vi "IMAQDevice.get_VideoModesAndAttributes.vi"(0 "i ref in":refnum<vi>, 5 "error in (no error)":errorcluster) -> (14 "i ref out":refnum<vi>, 16 "Video Modes":T3(array[cluster]), 17 "Attribute Information":T2(array[cluster]), 18 "Attribute Names":string[](array[string]), 19 "error out":errorcluster)   [LabVIEW 2014, in "IMAQDevice.lvlib"]
doc: "This VI reads back information from the camera.\n\nLicense Agreement for this software:\n\nCopyright (C)\nGesellschaft für Schwerionenforschung, GSI\nPlanckstr. 1\n64291 Darmstadt\nGermany\n\nContact: D.Beck@gsi.de \n\nThis program is free software; you can redistribute it and/or modify it under the terms of the \nGNU General Public License as published by the Free Software Foundation; either version 2 of \nthe license, or (at your option) any later version.\n\nThis program is distributed in the hope that it will be useful, but WITHOUT ANY WARRANTY; \nwithout even the implied warranty of MERCHANTABILITY or FITNESS FOR A PARTICULAR PURPOSE. See the GNU General License for more details (http://www.gnu.org).\n\nGesellschaft für Schwerionenforschung, GSI\nPlanckstr. 1, 64291 Darmstadt, Germany\nFor all questions and ideas contact: M.Richter@gsi.de, H.Brand@gsi.de or D.Beck@gsi.de.\nLast update: 16-JUN-2004"
uses:
  IMAQDevice.lvlib
  CSlibraries-extern/HGF/HGF_LVC/HGF_IMAQ/HGF_IMAQDevice/HGF_IMAQDevice.lvclass
  <vilib>/vision/driver/IMAQdx.llb/IMAQdx Attribute Type.ctl
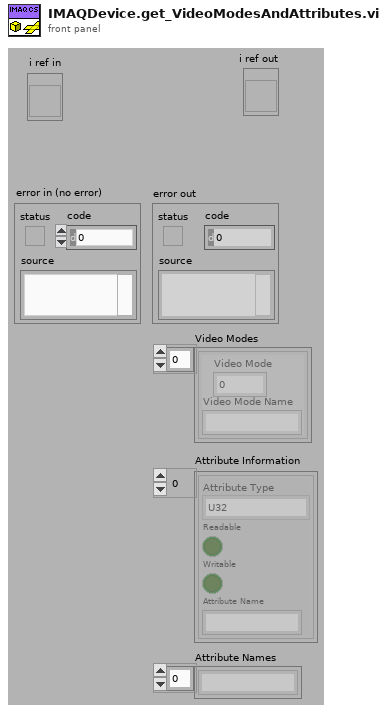
[diagram p1: front panel]
types:
  T1 = typedef "NI_Vision_Acquisition_Software.lvlib/IMAQdx Attribute Type.ctl" = enum32{"U32", "I64", "DBL", "String", "Enum", "Bool", "Command"}
  T2 = cluster{"Attribute Type":T1, "Readable":bool, "Writable":bool, "Attribute Name":string}[]
  T3 = cluster{"Video Mode":u32, "Video Mode Name":string}[]
  T4 = typedef "IMAQDevice.lvlib/IMAQDevice.i attribute.ctl" = cluster{"HGF_IMAQ.lvlib:HGF_IMAQDevice.lvclass":refnum<class "HGF_IMAQDevice.lvclass">, "Image":T5, "TimeStampID":i32, "Image IDs":i32[], "NumberOfImagesID":i32, "JPEG?":bool, "JPEGID":i32, "JPEG_ImageID":i32, "TriggerModeID":i32, "OffsetFromLeft":i32, "OffsetFromTop":i32, "HorizontalPixelPerMm":dbl, "VerticalPixelPerMm":dbl, "Grid":cluster{"1":cluster{i32, i32}, "2":cluster{i32, i32}, "3":cluster{i32, i32}, "4":cluster{i32, i32}}, "GridR":cluster{"1":cluster{dbl, dbl}, "2":cluster{dbl, dbl}, "3":cluster{dbl, dbl}, "4":cluster{dbl, dbl}}, "CameraTypeID":i32, "CameraInfos":cluster{"Camera Name-Array":string[], "own Camera Type":string}, "TakeMeasurement?":bool, "TriggerArmedID":i32, "Mirroring":i16, "Rotation":dbl}
  T5 = typedef "IMAQ Image.ctl" = refnum<image>
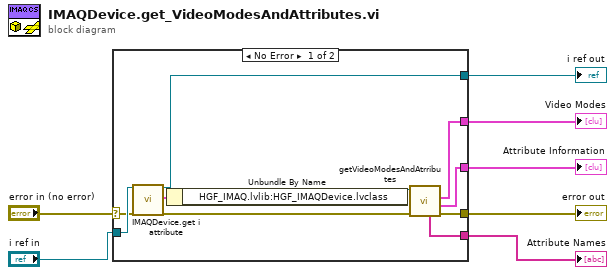
[diagram p0: block diagram]
diagram:
  n1 = case shown="No Error" "error in (no error)" {
    selector: "error in (no error)" -> [w16 w19]
    tunnel: "i ref in" -> [w17 w18]
    tunnel: [w10 w19] -> w5
    tunnel: [w14 w18] -> w4
    tunnel: [w11 _] -> w3
    tunnel: [w9 _] -> w2
    tunnel: [w8 _] -> w1
    frame No Error {
      n2 = call "IMAQDevice.get i attribute.vi"("i ref in"=w17, "error in (no error)"=w16) -> ("i ref out"=w14:refnum<vi>, "i attribute"=w15:T4, "error out"=w13:errorcluster)  [unwired: 15 in]
      n3 = Unbundle By Name(w15) -> ("HGF_IMAQ.lvlib:HGF_IMAQDevice.lvclass"=w12:refnum<class "HGF_IMAQDevice.lvclass">)
      n4 = call "getVideoModesAndAtrributes.vi"("error in (no error)"=w13, "HGF_IMAQDevice in"=w12) -> ("error out"=w10:errorcluster, "Attribute Information"=w9:T2, "Video Modes"=w11:T3, "Attribute Names"=w8:string[])  [unwired: 5 in, 1 out]
    }
    frame Error {
    }
  }
  "i ref out" <- w4
  "error out" <- w5
  "Video Modes" <- w3
  "Attribute Information" <- w2
  "Attribute Names" <- w1
